vi "Save Image.vi"(5 "Archive":bool, 7 "Dispose":bool, 8 "error in":errorcluster, 10 "Image in":T1, 11 "Config Manager in":refnum<class "Config Manager.lvclass">) -> (0 "error out":errorcluster, 2 "Image out":T1, 3 "Config Manager out":refnum<class "Config Manager.lvclass">)   [LabVIEW 2017, in "Config Manager.lvclass"]
uses:
  Config Manager.lvclass
  <vilib>/vision/Image Controls.llb/IMAQ Image.ctl
  Config Manager.lvclass/Config Manager.ctl
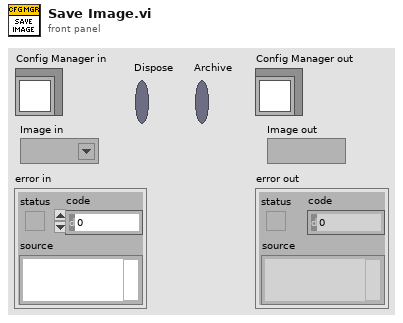
[diagram p1: front panel]
types:
  T1 = typedef "IMAQ Image.ctl" = refnum<image>
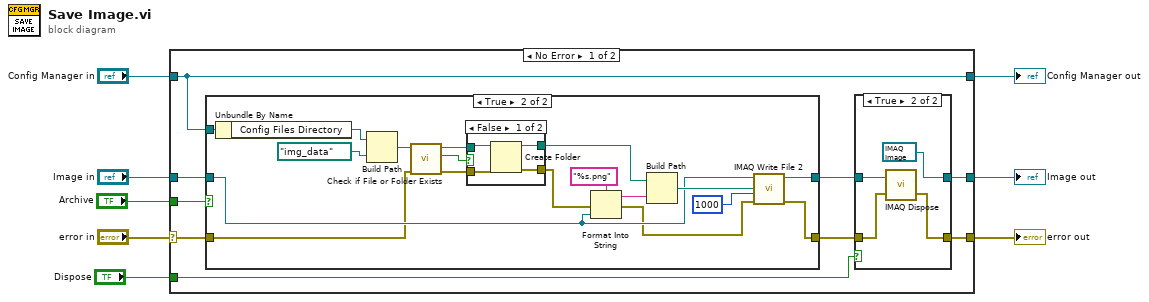
[diagram p0: block diagram]
diagram:
  n1 = case shown="No Error" "error in" {
    selector: "error in" -> [w14 w52]
    tunnel: [w9 w52] -> w7
    tunnel: [w17 w51] -> w5
    tunnel: "Config Manager in" -> [w17 w51]
    tunnel: "Image in" -> [w16 w50]
    tunnel: [w10 w50] -> w3
    tunnel: "Archive" -> [w15 _]
    tunnel: "Dispose" -> [w11 _]
    frame No Error {
      n2 = case shown="True" w15 {
        tunnel: w17 -> [_ w43]
        tunnel: w16 -> [w25 w33]
        tunnel: [w25 w31] -> w12
        tunnel: w14 -> [w24 w30]
        tunnel: [w24 w26] -> w13
        frame False {
        }
        frame True {
          n3 = Unbundle By Name(w43) -> ("Config Files Directory"=w42:path)
          n4 = Build Path(base path=w42, name or relative path=path "img_data" ("path")) -> (appended path=w40:path)
          n5 = call <vilib>:"Check if File or Folder Exists.vi"("error in (no error)"=w30, "path"=w40) -> ("error out"=w29:errorcluster, "file or folder exists?"=w38:bool, "dup path"=w37:path)  [unwired: 7 in]
          n6 = case shown="False" w38 {
            tunnel: w37 -> [w47 w49]
            tunnel: [w46 w49] -> w35
            tunnel: w29 -> [w45 w48]
            tunnel: [w44 w48] -> w28
            frame False {
              n7 = Create Folder(path (use dialog)=w47, error in=w45) -> (created path=w46:path, error out=w44:errorcluster)  [unwired: 1 in, 1 out]
            }
            frame True {
            }
          }
          n8 = Format Into String(format string="%s.png", error in=w28, w33) -> (resulting string=w39:string, error out=w27:errorcluster)  [unwired: 1 in]
          n9 = Build Path(base path=w35, name or relative path=w39) -> (appended path=w34:path)
          n10 = call-poly "IMAQ Write File 2"("error in (no error)"=w27, "Image Quality"=u32 1000, "File Path"=w34, "Image"=w33) -> ("error out"=w26:errorcluster, "Image Out (duplicate)"=w31:T1)  [unwired: 6 in]
        }
      }
      n11 = case shown="True" w11 {
        tunnel: w13 -> [w18 w21]
        tunnel: w12 -> [w19 w23]
        tunnel: [w19 T1 refnum ("Image in")] -> w10
        tunnel: [w18 w20] -> w9
        frame False {
        }
        frame True {
          n12 = call "IMAQ Dispose"("Image"=w23, "error in (no error)"=w21) -> ("error out"=w20:errorcluster)  [unwired: 4 in]
        }
      }
    }
    frame Error {
    }
  }
  "error out" <- w7
  "Config Manager out" <- w5
  "Image out" <- w3
